vi "SnoAutonomousMode.vi"() -> ()   [LabVIEW 2013]
uses:
  <vilib>/Utility/file.llb/Read From Spreadsheet File (string).vi
  Robot Global Data.vi
  <vilib>/Rock Robotics/WPI/RobotDrive/WPI_RobotDriveGetSetRefNum.vi
panel:
  out "Robot Driving":bool
  out "Delay Seconds":dbl
  out "Drive Time Velocity":dbl
  out "Drive Distance Velocity":dbl
  out "Time For Drive":dbl
  out "Dleay (milliseconds)":u32
  out "Drive Distance":dbl
  out "Degrees for Turn":i32
  out "Command Name":string
  out "all rows":string[][](array[string])
  out "Angular Rate":dbl
  out "Angle":dbl
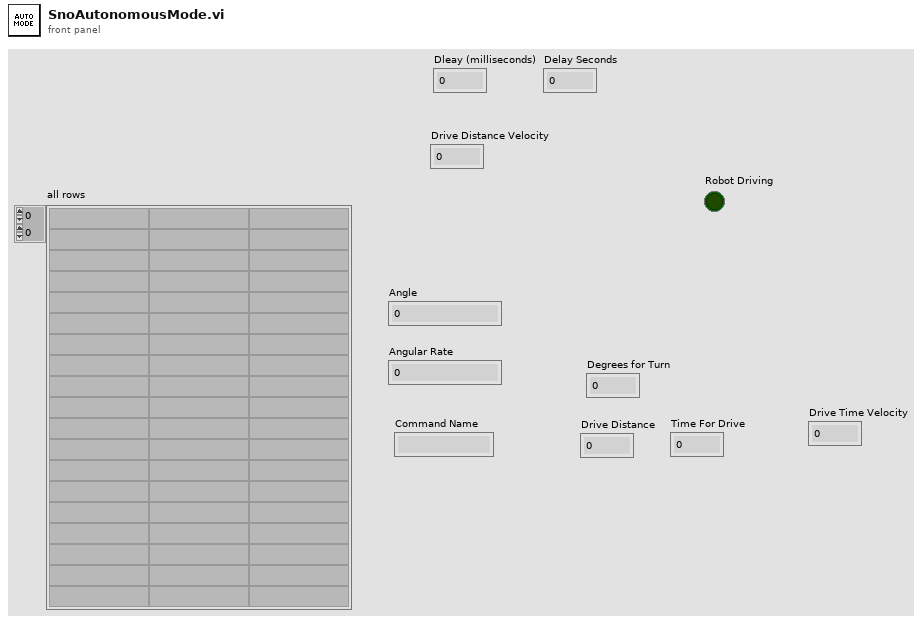
[diagram p1: front panel]
types:
  T1 = typedef "WPI_GyroDevRef.ctl" = cluster{"DevStatus":errorcluster, "Analog Module":T2, "Analog Channel":T3, "Offset":dbl, "Gain (VoltsPerDegree/Second)":dbl}
  T2 = typedef "FPGA_TypedefAnalogModule.ctl" = enum16{"Analog Module 1", "Analog Module 2"}
  T3 = typedef "FPGA_AIChannel.ctl" = enum8{"AI 1", "AI 2", "AI 3", "AI 4", "AI 5", "AI 6", "AI 7", "AI 8", "Invalid"}
  T4 = typedef "WPI_DriverStationLCDLCDLine.ctl" = enum16{"Main - Line 1", "User - Line 2", "User - Line 3", "User - Line 4", "User - Line 5", "User - Line 6"}
  T5 = typedef "WPI_RobotDriveDevRef.ctl" = cluster{"DevStatus":errorcluster, "Motors[]":T6[], "Square Inputs":bool, "Max Output":dbl, "Isochronous":bool}
  T6 = typedef "WPI_MotorControlDeviceRef.ctl" = cluster{"DeviceStatus":errorcluster, "Type":enum16{"PWM", "CAN"}, "PWM":cluster{"Digital Module":T7, "PWM Channel":T8, "DeadBand":T9}, "CAN":cluster{"Device Number":u8, "Control Mode":T10, "Semaphore":T11, "Max Vout":dbl}, "Invert":bool, "TransformRef":T12, "InvTransformRef":T12}
  T7 = typedef "FPGA_TypedefDigitalModule.ctl" = enum16{"Digital Module 1", "Digital Module 2"}
  T8 = typedef "FPGA_DIOPWMChannel.ctl" = enum8{"PWM 1", "PWM 2", "PWM 3", "PWM 4", "PWM 5", "PWM 6", "PWM 7", "PWM 8", "PWM 9", "PWM 10", "Invalid"}
  T9 = typedef "WPI_PWMDeadband.ctl" = cluster{"Name":string, "maxPositivePwm":i32, "minPositivePwm":i32, "centerPwm":i32, "maxNegativePwm":i32, "minNegativePwm":i32, "angularRange":u16}
  T10 = typedef "WPI_CANJaguar_ControlMode.ctl" = enum8{"Percent VBus", "Current", "Speed", "Position", "Voltage"}
  T11 = typedef "Semaphore RefNum" = refnum<k1>
  T12 = typedef "WPI_PWMTransform_ConPane.ctl" = refnum<vi>
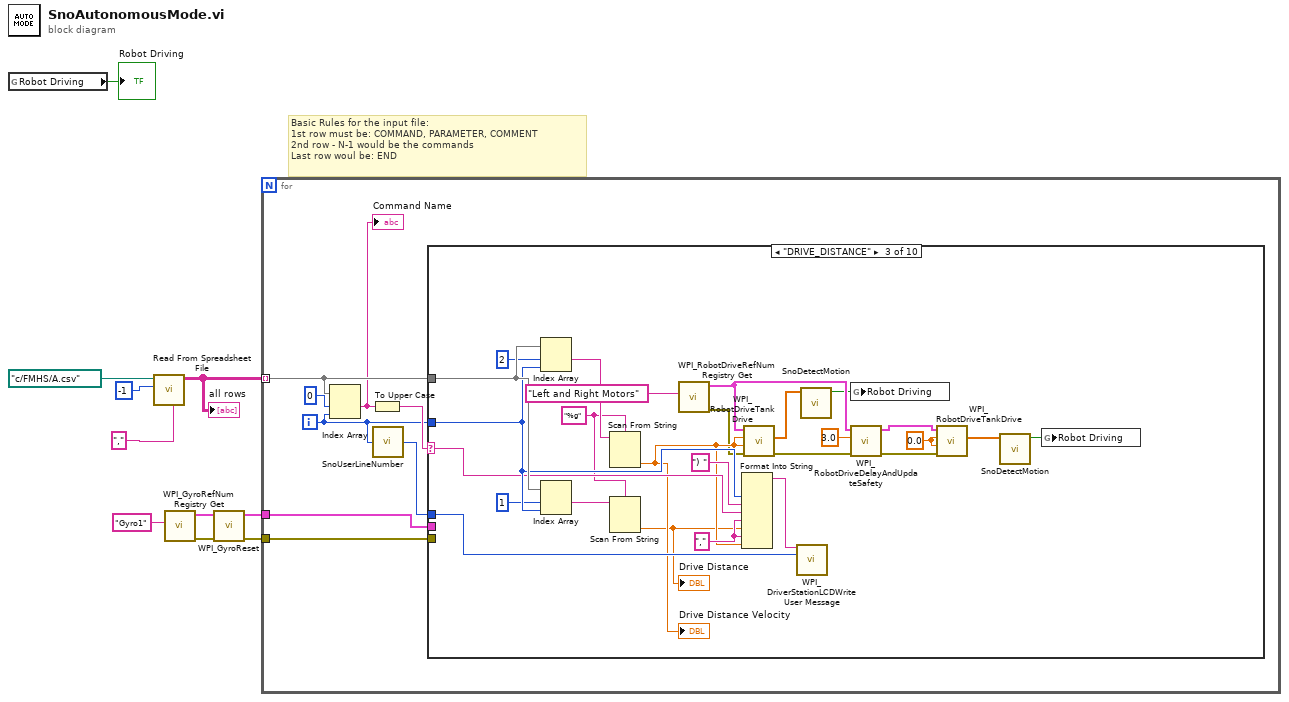
[diagram p0: block diagram]
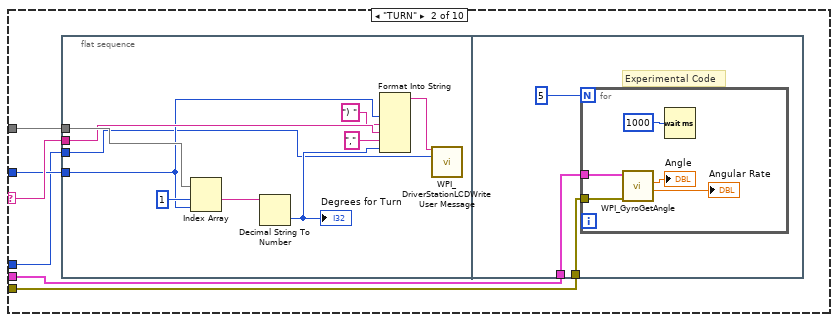
[diagram p3: hidden frame]
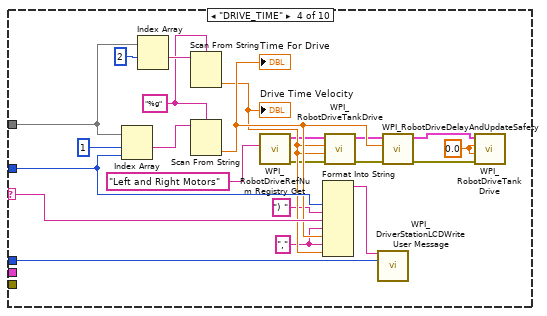
[diagram p4: hidden frame]
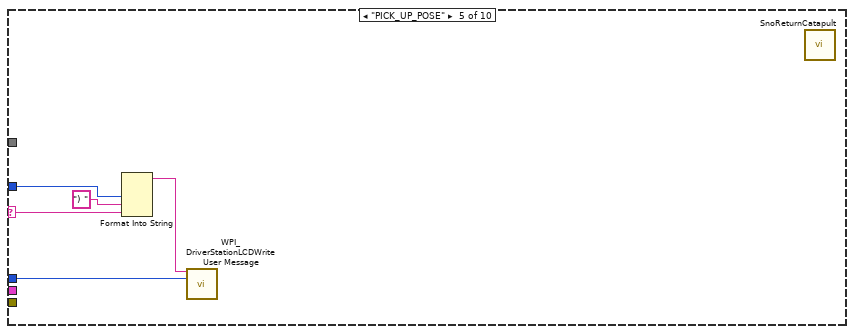
[diagram p5: hidden frame]
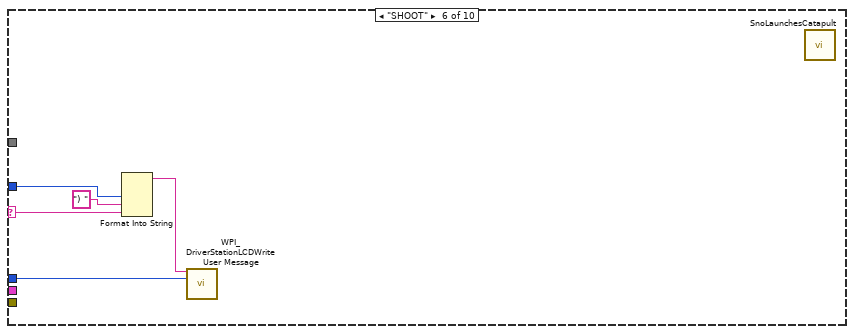
[diagram p6: hidden frame]
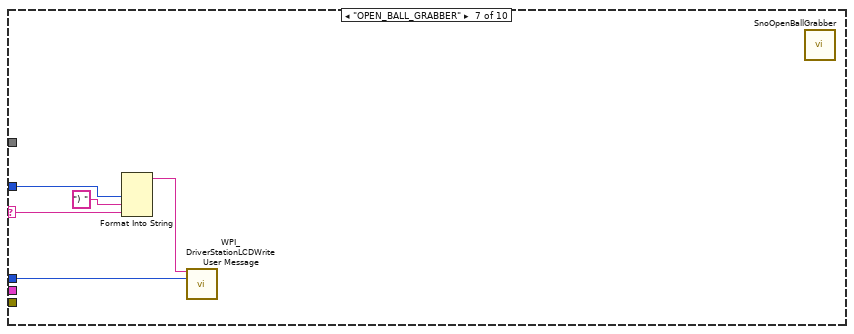
[diagram p7: hidden frame]
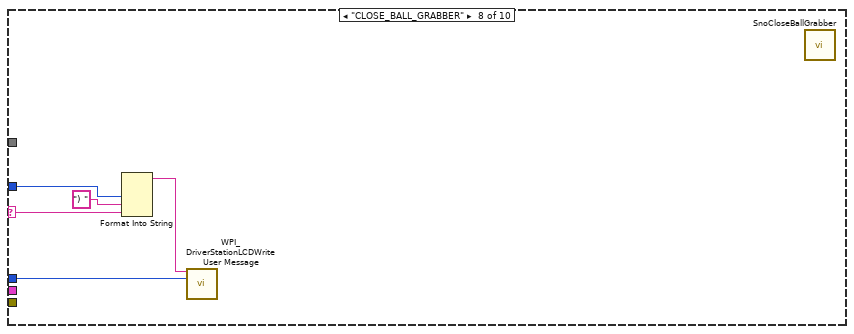
[diagram p8: hidden frame]
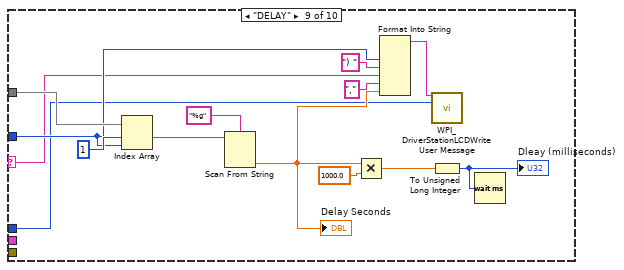
[diagram p9: hidden frame]
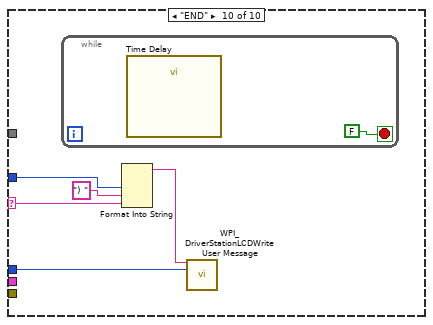
[diagram p10: hidden frame]
diagram:
  # "Basic Rules for the input file:\n1st row must be: COMMAND, PARAMETER, COMMENT\n2nd row - N-1 would be the commands\nLast row woul be: END"
  n1 = global read "Robot Global Data.vi" "Robot Driving"() -> (→"Robot Driving":bool)
  n2 = call-poly <vilib>:"Read From Spreadsheet File.vi"("delimiter (\\t)"="," ("delimiter (\\t)"), "number of rows (all:-1)"=-1, "file path (dialog if empty)"=path "c:/FMHS/A.csv" ("Simulator Script Name")) -> ("all rows"=w6:string[][])  [unwired: 4 in, 4 out]
  "all rows" <- w6
  n3 = call <vilib>:"WPI_GyroRefNum Registry Get.vi"("refnum name"="Gyro1") -> ("error out"=w8:errorcluster, "GyroDevRef"=w9:T1)  [unwired: 9 in]
  n4 = call <vilib>:"WPI_GyroReset.vi"("error in (no error)"=w8, "GyroDevRef"=w9) -> ("error out"=w3:errorcluster, "GyroDevRef"=w4:T1)  [unwired: 8 in]
  n5 = for {
    tunnel: w6 -> [w17] mode=indexing
    tunnel: w4 -> [w16]
    tunnel: w3 -> [w15]
    i -> [w12]
    n6 = Index Array(array=w17, index #1=0 ("index"), index #2=w12) -> (element #1=w13:string)  [unwired: 1 out]
    "Command Name" <- w13
    n7 = To Upper Case(1:w13) -> (0:w14:string)
    n8 = call "SnoUserLineNumber.vi"("Numeric"=w12) -> ("line"=w11:T4)
    n9 = case shown="\"DRIVE_DISTANCE\"" w14 {
      selector: w14 -> [_ w21 w66 w88 w92 w97 w102 w107 w116 w126]
      tunnel: w17 -> [_ w24 w68 w90 _ _ _ _ w124 _]
      tunnel: w12 -> [_ w20 w67 w89 w93 w98 w103 w108 w117 w127]
      tunnel: w16 -> [_ w23 _ _ _ _ _ _ _ _]
      tunnel: w15 -> [_ w22 _ _ _ _ _ _ _ _]
      tunnel: w11 -> [_ w19 w65 w87 w91 w96 w101 w106 w111 w125]
      frame "COMMAND", Default {
      }
      frame "TURN" {
        n10 = flat-sequence {
          tunnel: w24 -> [w33]
          tunnel: w20 -> [w27]
          tunnel: w21 -> [w28]
          tunnel: w19 -> [w25]
          tunnel: w23 -> [w36]
          tunnel: w22 -> [w35]
          frame #0 {
            n11 = Index Array(array=w33, index #1=1 ("index"), index #2=w27) -> (element #1=w34:string)  [unwired: 1 out]
            n12 = Decimal String To Number(string=w34) -> (number=w30:i32)  [unwired: 2 in, 1 out]
            "Degrees for Turn" <- w30
            n13 = Format Into String(w27, ") ", w28, ",", w30) -> (resulting string=w31:string)  [unwired: 3 in, 1 out]
            n14 = call <vilib>:"WPI_DriverStationLCDWrite User Message.vi"("line text"=w31, "line"=w25) -> ()  [unwired: 13 in, 1 out]
          }
          frame #1 {
            # "Experimental Code"
            n15 = for {
              N: 5 -> [_]
              tunnel: w36 -> [w39]
              tunnel: w35 -> [w38]
              n16 = call <vilib>:"WPI_GyroGetAngle.vi"("error in (no error)"=w38, "GyroDevRef"=w39) -> ("Angular Rate"=→"Angular Rate":dbl, "Angle"=→"Angle":dbl)  [unwired: 6 in, 2 out]
              n17 = Wait (ms)(milliseconds to wait=u32 1000) -> ()  [unwired: 1 out]
            }
          }
        }
      }
      frame "DRIVE_DISTANCE" {
        w51 = ","
        w46 = "%g" ("format string")
        w64 = 0.0 ("Left axis value")
        n18 = Index Array(array=w68, index #1=2 ("index"), index #2=w67) -> (element #1=w53:string)  [unwired: 1 out]
        n19 = Index Array(array=w68, index #1=1 ("index"), index #2=w67) -> (element #1=w47:string)  [unwired: 1 out]
        n20 = Scan From String(format string=w46, input string=w53) -> (output 1=w50:dbl)  [unwired: 3 in, 3 out]
        "Drive Distance Velocity" <- w50
        n21 = Scan From String(format string=w46, input string=w47) -> (output 1=w45:dbl)  [unwired: 3 in, 3 out]
        "Drive Distance" <- w45
        n22 = call <vilib>:"WPI_RobotDriveRefNum Registry Get.vi"("refnum name"="Left and Right Motors") -> ("error out"=w48:errorcluster, "RobotDriveDevRef"=w58:T5)  [unwired: 1 in, 8 out]
        n23 = Format Into String(w67, ") ", w66, w51, w45, w51, w50) -> (resulting string=w49:string)  [unwired: 3 in, 1 out]
        n24 = call <vilib>:"WPI_RobotDriveTankDrive.vi"("error in (no error)"=w48, "Right axis value"=w50, "Left axis value"=w50, "RobotDriveDevRef"=w58) -> ("error out"=w57:errorcluster, "Motor Values"=w44:dbl[])  [unwired: 5 in, 1 out]
        n25 = call <vilib>:"WPI_DriverStationLCDWrite User Message.vi"("line text"=w49, "line"=w65) -> ()  [unwired: 13 in, 1 out]
        n26 = call "SnoDetectMotion.vi"("Motor Values"=w44) -> ("Boolean"=w43:bool)  [unwired: 10 in]
        n27 = global write "Robot Global Data.vi" "Robot Driving"(w43) -> ()
        n28 = call <vilib>:"WPI_RobotDriveDelayAndUpdateSafety.vi"("error in (no error)"=w57, "Delay (s)"=3.0, "RobotDriveDevRef"=w58) -> ("error out"=w62:errorcluster, "RobotDriveDevRef 2"=w63:T5)  [unwired: 7 in]
        n29 = call <vilib>:"WPI_RobotDriveTankDrive.vi"("error in (no error)"=w62, "Right axis value"=w64, "Left axis value"=w64, "RobotDriveDevRef"=w63) -> ("Motor Values"=w60:dbl[])  [unwired: 5 in, 2 out]
        n30 = call "SnoDetectMotion.vi"("Motor Values"=w60) -> ("Boolean"=w61:bool)  [unwired: 10 in]
        n31 = global write "Robot Global Data.vi" "Robot Driving"(w61) -> ()
      }
      frame "DRIVE_TIME" {
        w71 = ","
        w69 = "%g" ("format string")
        w86 = 0.0 ("Left axis value")
        n32 = Index Array(array=w90, index #1=1 ("index"), index #2=w89) -> (element #1=w70:string)  [unwired: 1 out]
        n33 = Index Array(array=w90, index #1=2 ("index")) -> (element #1=w74:string)  [unwired: 1 in, 1 out]
        n34 = Scan From String(format string=w69, input string=w74) -> (output 1=w82:dbl)  [unwired: 3 in, 3 out]
        "Drive Time Velocity" <- w82
        n35 = Scan From String(format string=w69, input string=w70) -> (output 1=w83:dbl)  [unwired: 3 in, 3 out]
        "Time For Drive" <- w83
        n36 = call <vilib>:"WPI_RobotDriveRefNum Registry Get.vi"("refnum name"="Left and Right Motors") -> ("error out"=w81:errorcluster, "RobotDriveDevRef"=w80:T5)  [unwired: 1 in, 8 out]
        n37 = Format Into String(w89, ") ", w88, w71, w83, w71, w82) -> (resulting string=w73:string)  [unwired: 3 in, 1 out]
        n38 = call <vilib>:"WPI_RobotDriveTankDrive.vi"("error in (no error)"=w81, "Right axis value"=w82, "Left axis value"=w82, "RobotDriveDevRef"=w80) -> ("error out"=w78:errorcluster, "RobotDriveDevRef"=w79:T5)  [unwired: 5 in, 1 out]
        n39 = call <vilib>:"WPI_DriverStationLCDWrite User Message.vi"("line text"=w73, "line"=w87) -> ()  [unwired: 13 in, 1 out]
        n40 = call <vilib>:"WPI_RobotDriveDelayAndUpdateSafety.vi"("error in (no error)"=w78, "Delay (s)"=w83, "RobotDriveDevRef"=w79) -> ("error out"=w84:errorcluster, "RobotDriveDevRef 2"=w85:T5)  [unwired: 7 in]
        n41 = call <vilib>:"WPI_RobotDriveTankDrive.vi"("error in (no error)"=w84, "Right axis value"=w86, "Left axis value"=w86, "RobotDriveDevRef"=w85) -> ()  [unwired: 5 in, 3 out]
      }
      frame "PICK_UP_POSE" {
        n42 = Format Into String(w93, ") ", w92) -> (resulting string=w95:string)  [unwired: 3 in, 1 out]
        n43 = call <vilib>:"WPI_DriverStationLCDWrite User Message.vi"("line text"=w95, "line"=w91) -> ()  [unwired: 13 in, 1 out]
        n44 = call "SnoReturnCatapult.vi"() -> ()  [unwired: 12 in]
      }
      frame "SHOOT" {
        n45 = Format Into String(w98, ") ", w97) -> (resulting string=w100:string)  [unwired: 3 in, 1 out]
        n46 = call <vilib>:"WPI_DriverStationLCDWrite User Message.vi"("line text"=w100, "line"=w96) -> ()  [unwired: 13 in, 1 out]
        n47 = call "SnoLaunchesCatapult.vi"() -> ()  [unwired: 12 in]
      }
      frame "OPEN_BALL_GRABBER" {
        n48 = Format Into String(w103, ") ", w102) -> (resulting string=w105:string)  [unwired: 3 in, 1 out]
        n49 = call <vilib>:"WPI_DriverStationLCDWrite User Message.vi"("line text"=w105, "line"=w101) -> ()  [unwired: 13 in, 1 out]
        n50 = call "SnoOpenBallGrabber.vi"() -> ()  [unwired: 1 in, 1 out]
      }
      frame "CLOSE_BALL_GRABBER" {
        n51 = Format Into String(w108, ") ", w107) -> (resulting string=w110:string)  [unwired: 3 in, 1 out]
        n52 = call <vilib>:"WPI_DriverStationLCDWrite User Message.vi"("line text"=w110, "line"=w106) -> ()  [unwired: 13 in, 1 out]
        n53 = call "SnoCloseBallGrabber.vi"() -> ()  [unwired: 1 in, 2 out]
      }
      frame "DELAY" {
        n54 = Index Array(array=w124, index #1=1 ("index"), index #2=w117) -> (element #1=w115:string)  [unwired: 1 out]
        n55 = Scan From String(format string="%g", input string=w115) -> (output 1=w113:dbl)  [unwired: 3 in, 3 out]
        "Delay Seconds" <- w113
        n56 = Multiply(x=w113, y=1000.0) -> (x*y=w121:dbl)
        n57 = Format Into String(w117, ") ", w116, ",", w113) -> (resulting string=w120:string)  [unwired: 3 in, 1 out]
        n58 = call <vilib>:"WPI_DriverStationLCDWrite User Message.vi"("line text"=w120, "line"=w111) -> ()  [unwired: 13 in, 1 out]
        n59 = To Unsigned Long Integer(number=w121) -> (unsigned 32bit integer=w112:u32)
        "Dleay (milliseconds)" <- w112
        n60 = Wait (ms)(milliseconds to wait=w112) -> ()  [unwired: 1 out]
      }
      frame "END" {
        n61 = while {
          stop <- FALSE stop-if-true
          n62 = call "Time Delay"() -> ()  [unwired: 11 in, 1 out]
        }
        n63 = Format Into String(w127, ") ", w126) -> (resulting string=w129:string)  [unwired: 3 in, 1 out]
        n64 = call <vilib>:"WPI_DriverStationLCDWrite User Message.vi"("line text"=w129, "line"=w125) -> ()  [unwired: 13 in, 1 out]
      }
    }
  }
